vi "MainNR.vi"(10 "JQMHStartup.lvclass":refnum<class "RQMHStartup.lvclass">, 11 "TesterModule in":refnum<class "Watchdog.lvclass">) -> ()   [LabVIEW 2024, in "Watchdog.lvclass"]
uses:
  Watchdog.lvclass
  JQMHCore/JQMHStartup/RQMHStartup.lvclass
  Watchdog.lvclass/Watchdog.ctl
  JQMHCore/Shared/JQMHShared.lvlib
  JQMHCore/Module/RQMHModule.lvclass
  C:/Github/JQMH/JQMHCore/Module/RQMHModule.lvclass
  C:/Github/JQMH/Watchdog/Watchdog.lvclass
panel:
  out "error out":errorcluster
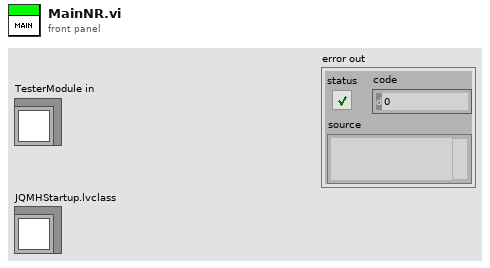
[diagram p1: front panel]
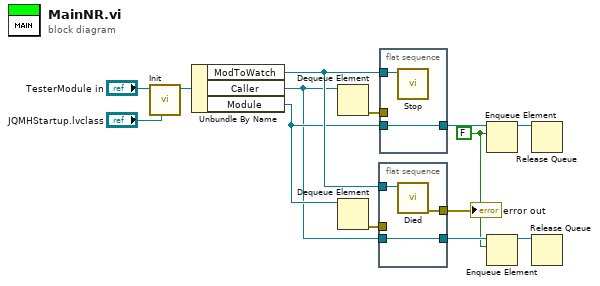
[diagram p0: block diagram]
diagram:
  w3 = FALSE ("element")
  n1 = call "Init.vi"("JQMHStartup.lvclass"="JQMHStartup.lvclass", "JQMHCore.lvclass"="TesterModule in") -> ("JQMHCore out"=w13:refnum<class "Watchdog.lvclass">)  [unwired: 5 in, 4 out]
  n2 = Unbundle By Name(w13) -> ("ModToWatch"=w10:refnum<class "RQMHModule.lvclass">, "Caller"=w4:refnum<queue>, "Module"=w9:refnum<queue>)
  n3 = Dequeue Element(queue=w4) -> (error out=w12:errorcluster)  [unwired: 2 in, 3 out]
  n4 = Dequeue Element(queue=w9) -> (error out=w11:errorcluster)  [unwired: 2 in, 3 out]
  n5 = flat-sequence {
    tunnel: w10 -> [w17]
    tunnel: w11 -> [_]
    tunnel: [w16] -> w5
    tunnel: w4 -> [w16]
    tunnel: [w15] -> w2
    frame #0 {
      n6 = call "Died.vi"("JQMHModule in"=w17) -> ("error out"=w15:errorcluster)  [unwired: 9 in, 1 out]
    }
  }
  n7 = flat-sequence {
    tunnel: w10 -> [w19]
    tunnel: w12 -> [_]
    tunnel: w9 -> [w18]
    tunnel: [w18] -> w8
    frame #0 {
      n8 = call "Stop.vi"("JQMHCore in"=w19) -> ()  [unwired: 10 in, 1 out]
    }
  }
  n9 = Enqueue Element(queue=w8, element=w3) -> (queue out=w7:refnum<queue>)  [unwired: 2 in, 2 out]
  n10 = Enqueue Element(queue=w5, element=w3) -> (queue out=w6:refnum<queue>)  [unwired: 2 in, 2 out]
  n11 = Release Queue(queue=w7) -> ()  [unwired: 2 in, 3 out]
  n12 = Release Queue(queue=w6) -> ()  [unwired: 2 in, 3 out]
  "error out" <- w2
